vi "ASDA-A2_Get Monitot Data.vi"(8 "error in":errorcluster, 11 "Buffer Data In":T1) -> (0 "error out":errorcluster, 2 "Data":i32[](array[numeric]), 3 "Buffer Data Out":T1)   [LabVIEW 2016]
uses:
  Data Def/ASDA-A2_Buffer Data.ctl
  Data Def/ASDA-A2_Read Register Data.ctl
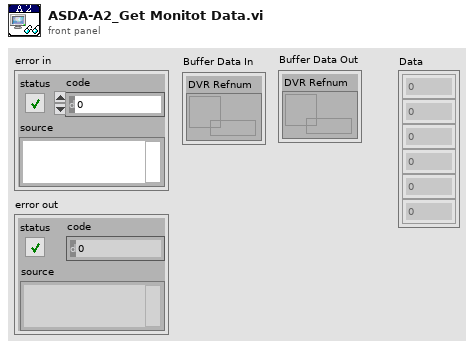
[diagram p1: front panel]
types:
  T1 = typedef "ASDA-A2_Buffer Data.ctl" = cluster{"DVR Refnum":refnum<data-value>}
  T2 = typedef "ASDA-A2_Read Register Data.ctl" = cluster{"Address":u16, "Count":u16, "Page":string, "Description":string}
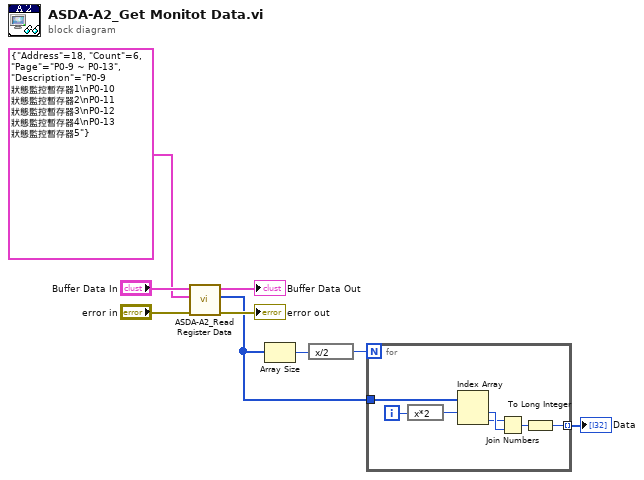
[diagram p0: block diagram]
diagram:
  n1 = call "ASDA-A2_Read Register Data.vi"("error in"="error in", "Read Register Data"=T2 {"Address"=18, "Count"=6, "Page"="P0-9 ~ P0-13", "Description"="P0-9   狀態監控暫存器1\nP0-10 狀態監控暫存器2\nP0-11 狀態監控暫存器3\nP0-12 狀態監控暫存器4\nP0-13 狀態監控暫存器5"}, "Buffer Data In"="Buffer Data In") -> ("error out"=→"error out":errorcluster, "Data"=w2:u16[], "Buffer Data Out"=→"Buffer Data Out":T1)  [unwired: 6 in]
  n2 = Array Size(array=w2) -> (size(s)=w4:i32)
  n3 = expression code="x/2"(w4) -> (w3:i32)
  n4 = for {
    N: w3 -> [_]
    tunnel: [w13] -> w1 mode=indexing
    tunnel: w2 -> [w12]
    i -> [w16]
    n5 = expression code="x*2"(w16) -> (w15:i32)
    n6 = Index Array(array=w12, index #1=w15) -> (element #1=w11:u16, element #2=w10:u16)  [unwired: 1 in]
    n7 = Join Numbers(hi=w10, lo=w11) -> ((hi.lo)=w14:u32)
    n8 = To Long Integer(number=w14) -> (32bit integer=w13:i32)
  }
  "Data" <- w1
